vi "mac_mem_accum_32bit_pipe.vi"(6 "sclr":bool, 9 "x_i":T2, 10 "readIndex":u8, 11 "Refnum in":refnum<k21>) -> (3 "s":T1=-1.0)   [LabVIEW 2017]
uses:
  x_qp_scalar.ctl
  xtype_scalar.ctl
  <vilib>/rvi/IPIntegrationNode/IPINode_Typedef/niFpgaIPINodeSupportedFamilies.ctl
  <vilib>/rvi/DataTransferAndStorage/Container/Common/niFpgaContainerExecOnDevCompGetState.vi
  <vilib>/rvi/Emulation/niFpgaEmulationIsFPGAContextNoSignature.vi
  <vilib>/rvi/DataTransferAndStorage/Container/Common/niFpgaContainerGetUniqueNameForEmu.vi
  <vilib>/rvi/Emulation/niFpgaProcessEmulError.vi
  <vilib>/rvi/Emulation/niFpgaSctlEmulationGetInTimedLoop.vi
  <vilib>/rvi/errors/nirviReportUnexpectedCaseInternalError (U32).vi
  <vilib>/rvi/Memory/Memory_Emulation/niFpgaMemoryEmulationCacheClearOnFirstRun.vi
  <vilib>/rvi/Memory/Memory_Emulation/nirvimemoryEmulationManagerCache_MakeExclusive.vi
  <vilib>/rvi/Memory/Memory_Emulation/niFpgaMemoryEmulationValidateCache.vi
  <vilib>/rvi/Memory/Memory_Emulation/nirvimemoryEmulationManagerCache_InsertValue.vi
  <vilib>/Utility/error.llb/Clear Errors.vi
  <vilib>/rvi/Memory/Memory_Emulation/nirvimemoryEmulationManagerCache_ReleaseExclusive.vi
  <vilib>/rvi/Memory/Memory_Emulation/nirvimemoryEmulationManagerCache_GetValue.vi
  <vilib>/rvi/Memory/Memory_Emulation/nirvimemoryEmulationManagerCache_SetValue.vi
  <vilib>/rvi/Emulation/niFpgaSctlEmulationResourceMgr.vi
  <vilib>/rvi/IPIntegrationNode/IPINode_Utilities/niFpgaIPINodeSimCore.vi
  <vilib>/rvi/DataTransferAndStorage/Container/XNode/niFpgaContainer.xnode
  <vilib>/rvi/Memory/Memory_Emulation/niFpgaMemoryEmulationRefIn.vi
  <vilib>/rvi/XilinxIP/XIPIN_XNode/niFpgaXIPIN.xnode
  mults_acums/mac01/Multiply_Accumulator_C1CFE835F5094677B11E60272D0552B5.dll
  <vilib>/rvi/IPIntegrationNode/IPINode_Xnode/niFpgaIPINode.xnode
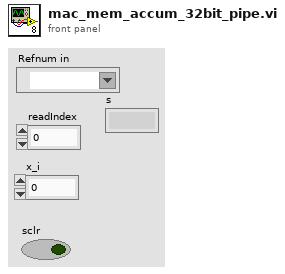
[diagram p1: front panel]
types:
  T1 = typedef "xtype_scalar.ctl" = fxp<+/-,32,6>
  T2 = typedef "x_qp_scalar.ctl" = fxp<+/-,32,6>
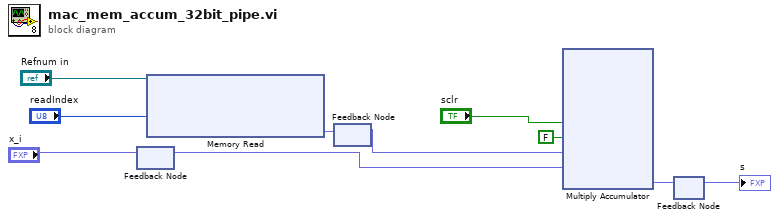
[diagram p0: block diagram]
diagram:
  n1 = feedback #1() -> (w7:T2)  [unwired: 1 in]
  n2 = feedback-in #1("x_i") -> ()
  n3 = xnode ("Memory Read")("Address"="readIndex", "Memory In"="Refnum in") -> ("Data"=w10:fxp<+/-,32,2>)  [unwired: 1 out]
  n4 = feedback #2() -> (w6:fxp<+/-,32,2>)  [unwired: 1 in]
  n5 = feedback-in #2(w10) -> ()
  n6 = xnode ("Multiply Accumulator")("sclr"="sclr", "bypass"=FALSE, "a"=w6, "b"=w7) -> ("s"=w2:fxp<+/-,32,8>)  [unwired: 1 in]
  n7 = feedback #3() -> (→"s":fxp<+/-,32,8>)  [unwired: 1 in]
  n8 = feedback-in #3(w2) -> ()
